vi "Any file exists -- V1.vi"(8 "Error In":errorcluster, 11 "Files":path[](array[path])) -> (0 "Error Out":errorcluster, 3 "Any file exists?":bool)   [LabVIEW 2021]
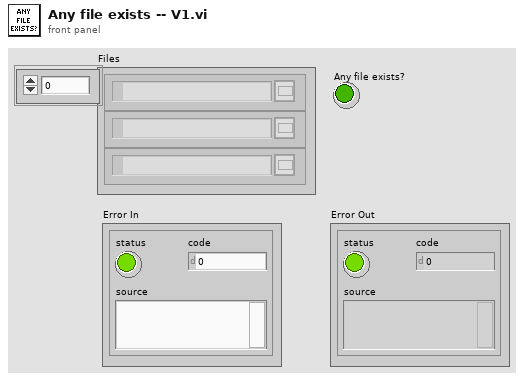
[diagram p1: front panel]
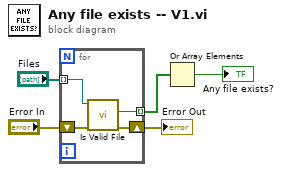
[diagram p0: block diagram]
diagram:
  n1 = for {
    tunnel: "Files" -> [w9] mode=indexing
    shift-right: [w6] -> w3
    shift-left: "Error In" -> [w7]
    tunnel: [w8] -> w2 mode=indexing
    n2 = call "Is Valid File.vi"("Error In"=w7, "File"=w9) -> ("Error Out"=w6:errorcluster, "Valid file"=w8:bool)  [unwired: 7 in, 1 out]
  }
  "Error Out" <- w3
  n3 = Or Array Elements(Boolean array=w2) -> (logical OR=→"Any file exists?":bool)
